vi "Write Header.vi"(8 "error in (no error)":errorcluster, 10 "Header":string, 11 "Update Header MSG in":refnum<class "Update Header MSG.lvclass">) -> (0 "error out":errorcluster, 3 "Update Header MSG out":refnum<class "Update Header MSG.lvclass">)   [LabVIEW 2017, in "File Library.lvlib" / "Update Header MSG.lvclass"]
uses:
  Update Header MSG.lvclass
  Update Header MSG.lvclass/Update Header MSG.ctl
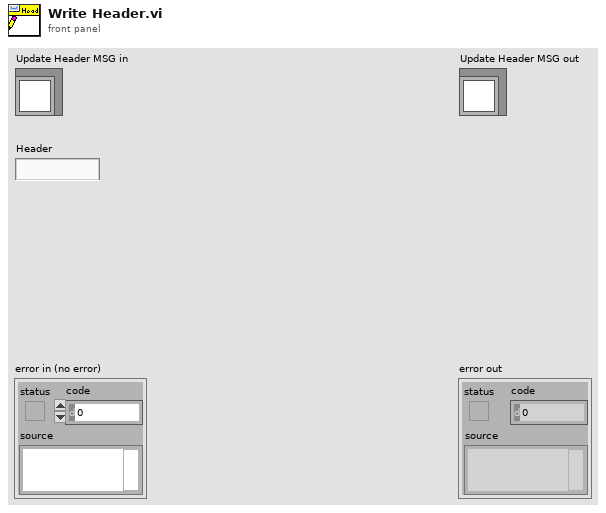
[diagram p1: front panel]
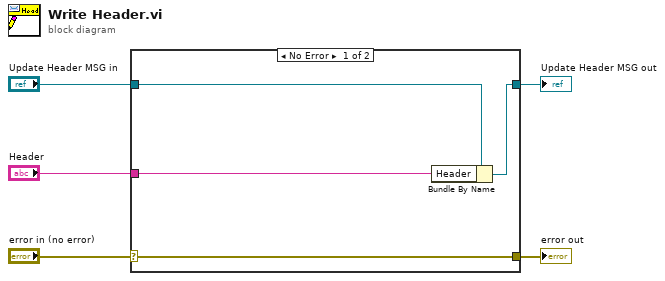
[diagram p0: block diagram]
diagram:
  n1 = case shown="No Error" "error in (no error)" {
    selector: "error in (no error)" -> [w9 w10]
    tunnel: [w9 w10] -> w4
    tunnel: [w7 w11] -> w2
    tunnel: "Update Header MSG in" -> [w8 w11]
    tunnel: "Header" -> [w6 _]
    frame No Error {
      n2 = Bundle By Name(cluster=w8, "Header"=w6) -> (w7:refnum<class "Update Header MSG.lvclass">)
    }
    frame Error {
    }
  }
  "error out" <- w4
  "Update Header MSG out" <- w2
